vi "Create New Report.vi"(8 "error in (no error)":errorcluster, 9 "Report Path":path, 11 "TestMonitor in":refnum<class "TestMonitor.lvclass">) -> (0 "error out":errorcluster, 3 "TestMonitor out":refnum<class "TestMonitor.lvclass">)   [LabVIEW 2018, in "TestMonitor.lvclass"]
uses:
  TestMonitor.lvclass
  TestMonitor.lvclass/TestMonitor.ctl
  <vilib>/Skyline/TestMonitor/Test Result/Create Test Result (Single).vi
  <vilib>/Skyline/TestMonitor/Test Result/NI SystemLink Test Result.lvclass
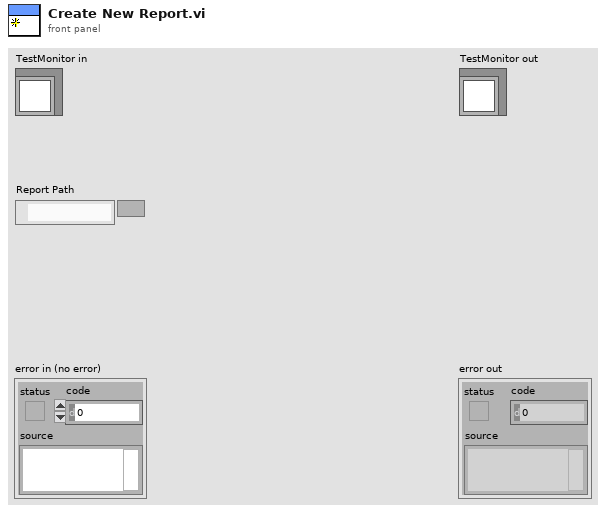
[diagram p1: front panel]
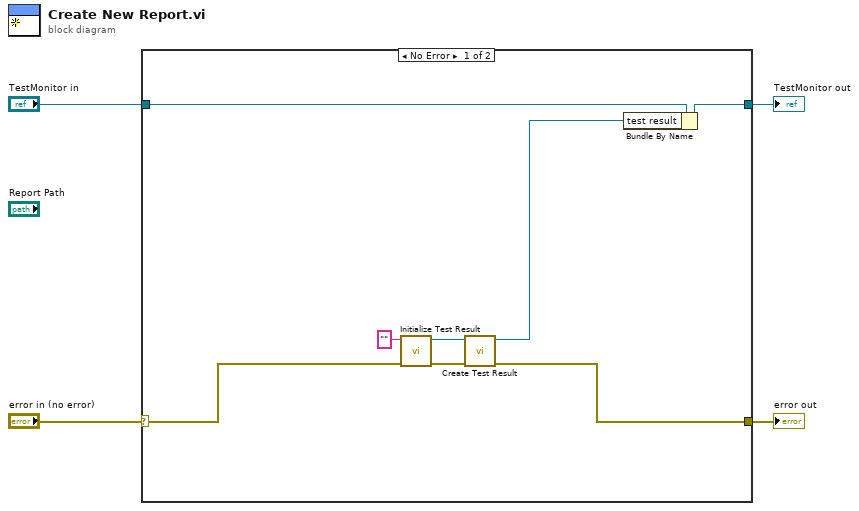
[diagram p0: block diagram]
diagram:
  n1 = case shown="No Error" "error in (no error)" {
    selector: "error in (no error)" -> [w9 w13]
    tunnel: [w8 w13] -> w4
    tunnel: [w7 w14] -> w2
    tunnel: "TestMonitor in" -> [w12 w14]
    frame No Error {
      n2 = call <vilib>:"Initialize Test Result.vi"("error in (no error)"=w9, "program name"="") -> ("error out"=w11:errorcluster, "test result"=w10:refnum<class "NI SystemLink Test Result.lvclass">)  [unwired: 8 in]
      n3 = call-poly <vilib>:"Create Test Result.vi"("error in (no error)"=w11, "test result out"=w10) -> ("error out"=w8:errorcluster, "test result out"=w6:refnum<class "NI SystemLink Test Result.lvclass">)  [unwired: 8 in]
      n4 = Bundle By Name(cluster=w12, "test result"=w6) -> (w7:refnum<class "TestMonitor.lvclass">)
    }
    frame Error {
    }
  }
  "error out" <- w4
  "TestMonitor out" <- w2
